vi "MatrixB_Tdep.vi"(0 "T-table String":string, 3 "Time Stamp":timestamp, 6 "Play Button":bool, 7 "Custom Folder":string, 8 "Settings":T2={"Ring 3"=1, "Ring 2"=4, "Fixed Current mkA"=0.5, "If yes, the current is:"=enum."Radio Selection 1", "Ressitance measurements?"=TRUE, "Commute DC current?"=FALSE} {"Ring 3" items=["1 kOhm", "10 kOhm", "100 kOhm", "1 Mohm", "10 mOhm"]; "Ring 2" items=["1 kOhm", "10 kOhm", "100 kOhm", "1 Mohm", "10 MOhm"]}, 9 "Instruments":T3={"Oscillator"=TRUE, "Addr 1 lock-in"=TRUE, "Addr 1 lock-in oop"=TRUE, "Addr 2 lock-in"=TRUE, "Addr 2 lock-in oop"=TRUE, "Addr 3 lock-in"=FALSE, "Addr 3 lock-in oop"=FALSE, "Voltage (Vk1)"=FALSE, "Current (Ik1)"=TRUE, "Voltage (Vk2)"=FALSE, "Current (Ik2)"=FALSE, "Voltage (Vk3)"=FALSE, "Current (Ik3)"=FALSE, "Channel 1 (Vnano1)  "=FALSE, "Channel 2 (Vnano1b)"=FALSE, "Channel 1 (Vnano2)   "=FALSE, "Channel 2 (Vnano2b)"=FALSE, "Thermometer 1 (T1)"=TRUE, "Magnetic Field (B)"=TRUE, "Capacitance (C) and Loss (L)"=FALSE}, 10 "BCluster":T4={"B1 (V)"=-1.0, "B2 (V)"=1.0, "Sweep rate, T/min"=0.5, "Time btw \npoints, sec"=1.0, "No-record rate, T/min"=0.5, "Full sweep?"=FALSE, "Odd confgurations"=TRUE} {"No-record rate, T/min" min=0.0 max=1.0 step=0.01 format="%_4f"; "B2 (V)" min=-4.0 max=4.0 step=0.1 format="%.1f"; "Time btw \npoints, sec" format="%.2f"; "Sweep rate, T/min" min=0.0 max=1.0 step=0.01 format="%_4f"; "B1 (V)" min=-4.0 max=4.0 step=0.1 format="%.1f"}, 11 "TCluster":T1={"Starting T (K)"=-1.0, "Final T (K)"=1.0, "Step (T)"=1.0, "Time for T stabilisation , min"=1.0, "Wait 1st point?"=FALSE, "At the end:"=TRUE} {"Final T (K)" min=-4.0 max=4.0 step=0.1 format="%.2f"; "Time for T stabilisation , min" format="%.2f"; "Step (T)" min=0.0 max=1.0 step=0.01 format="%_4f"; "Starting T (K)" min=-4.0 max=4.0 step=0.1 format="%.2f"}) -> ()   [LabVIEW 2017]
uses:
  <vilib>/Utility/file.llb/Read From Spreadsheet File (DBL).vi
panel:
  in  "No record Vg rate (V/min)":dbl=150.0
  in  "Voltage (sourse)":dbl
  out "Communication":string
  out "B Array":dbl[](array[numeric])
  out "Experiment ends at:":string
  out "Hours":dbl format="%.1f"
  out "Estimated time of experiment:":i16
  out "ArraySens":i8[](array[numeric])
  out "ArrayOsc":dbl[](array[numeric])
  out "# of configurations":i8
  out "Large Array":bool[][][](array[boolean])
  out "Contact configuration file (*.conf)":path
  # "1"
  # "hours"
  # "min.="
  # "Values of T can be also entered as the table by copying\nand pasting a column of numbers in a \"T table\" string at the \nfar right side of this window."
  # "Lock-in Amplifiers"
  # "Temperature"
  # "SourceMeters"
  # "Nanovoltmeters"
  # "Main"
  # "(not recommended, too slow)"
  # "Magnetic Field"
  # "Capacitance & Loss"
  # "(not recommended, too slow)"
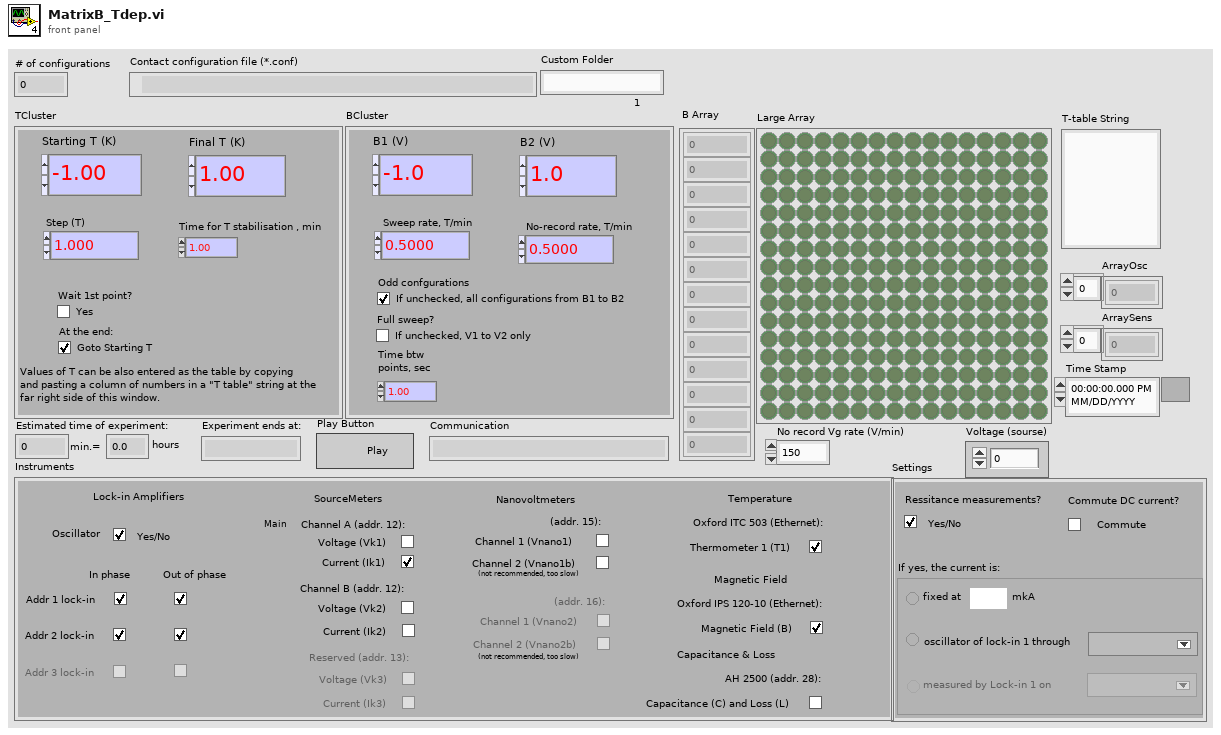
[diagram p1: front panel]
types:
  T1 = cluster{"Starting T (K)":dbl, "Final T (K)":dbl, "Step (T)":dbl, "Time for T stabilisation , min":dbl, "Wait 1st point?":bool, "At the end:":bool}
  T2 = cluster{"Ring 3":u16, "Ring 2":u16, "Fixed Current mkA":dbl, "If yes, the current is:":enum32{"Radio Selection 1", "Radio Selection 2", "Radio Selection 3"}, "Ressitance measurements?":bool, "Commute DC current?":bool}
  T3 = cluster{"Oscillator":bool, "Addr 1 lock-in":bool, "Addr 1 lock-in oop":bool, "Addr 2 lock-in":bool, "Addr 2 lock-in oop":bool, "Addr 3 lock-in":bool, "Addr 3 lock-in oop":bool, "Voltage (Vk1)":bool, "Current (Ik1)":bool, "Voltage (Vk2)":bool, "Current (Ik2)":bool, "Voltage (Vk3)":bool, "Current (Ik3)":bool, "Channel 1 (Vnano1)  ":bool, "Channel 2 (Vnano1b)":bool, "Channel 1 (Vnano2)   ":bool, "Channel 2 (Vnano2b)":bool, "Thermometer 1 (T1)":bool, "Magnetic Field (B)":bool, "Capacitance (C) and Loss (L)":bool}
  T4 = cluster{"B1 (V)":dbl, "B2 (V)":dbl, "Sweep rate, T/min":dbl, "Time btw \npoints, sec":dbl, "No-record rate, T/min":dbl, "Full sweep?":bool, "Odd confgurations":bool}
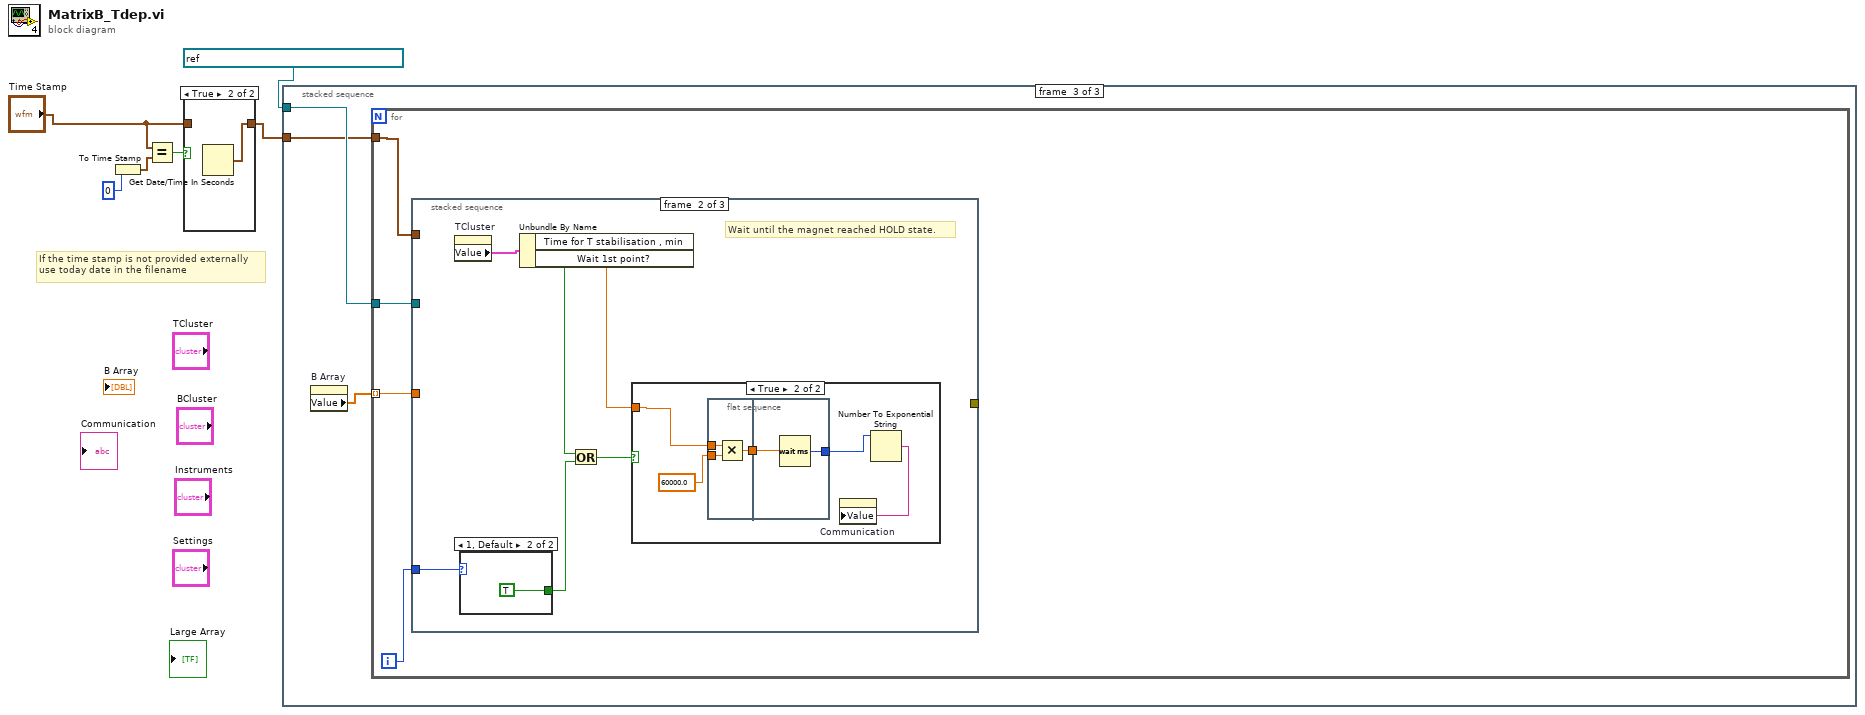
[diagram p0: block diagram]
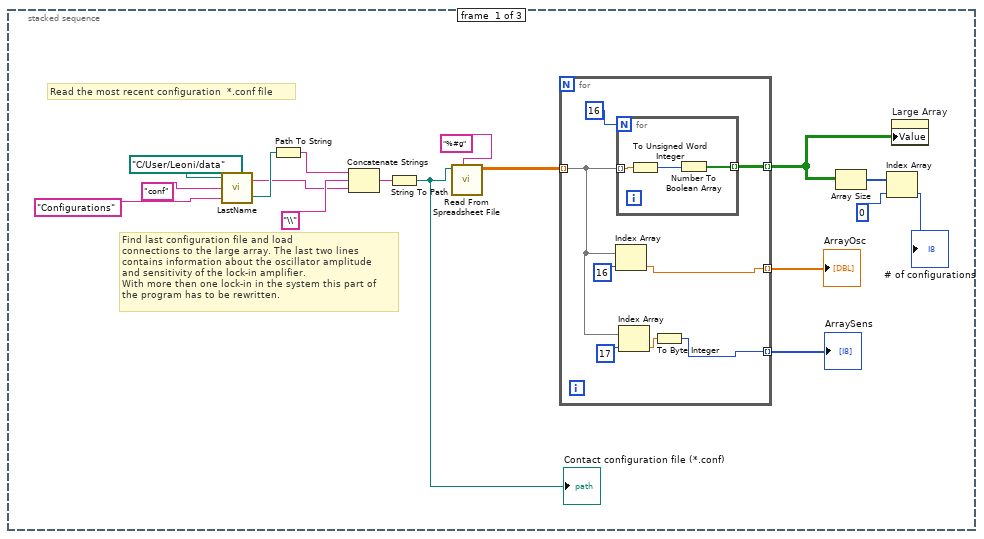
[diagram p3: hidden frame]
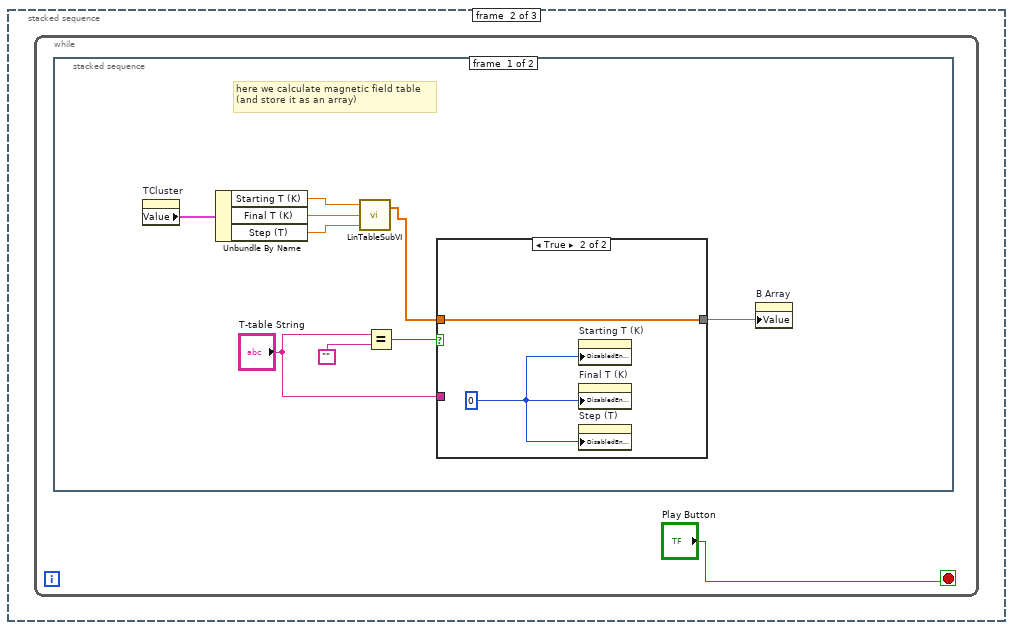
[diagram p4: hidden frame]
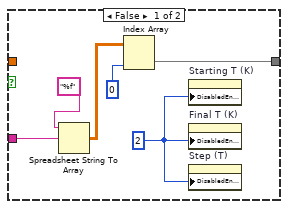
[diagram p5: hidden frame]
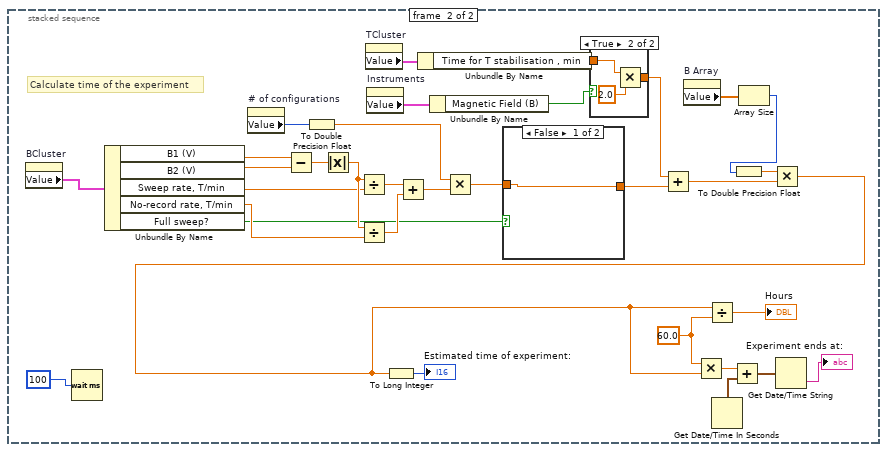
[diagram p6: hidden frame]
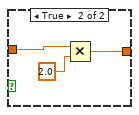
[diagram p8: hidden frame]
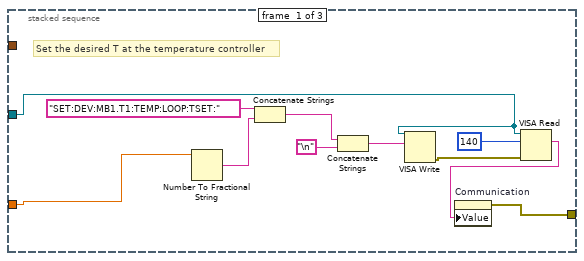
[diagram p9: hidden frame]
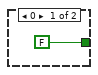
[diagram p11: hidden frame]
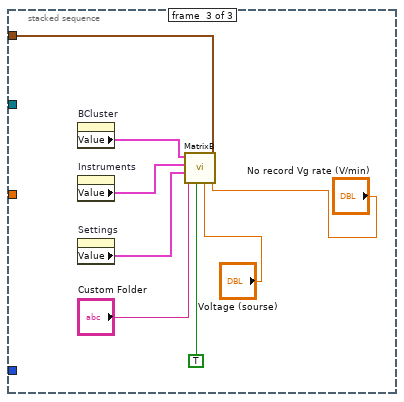
[diagram p12: hidden frame]
diagram:
  # "If the time stamp is not provided externally\nuse today date in the filename"
  n1 = To Time Stamp(1:0) -> (0:w5:timestamp)
  n2 = Equal?(x="Time Stamp", y=w5) -> (x = y?=w4:bool)
  n3 = case shown="True" w4 {
    tunnel: "Time Stamp" -> [w7 _]
    tunnel: [w7 w8] -> w2
    frame False {
    }
    frame True {
      n4 = Get Date/Time In Seconds() -> (seconds since 1Jan1904=w8:timestamp)
    }
  }
  n5 = stacked-sequence {
    tunnel: w2 -> [_ _ w96]
    tunnel: refnum<visa-resource-name> "TCPIP0::192.168.128.2::7020::SOCKET" ("VISA resource name") -> [_ _ w98]
    frame #0 {
      # "Read the most recent configuration  *.conf file"
      # "Find last configuration file and load \nconnections to the large array. The last two lines \ncontains information about the oscillator amplitude\nand sensitivity of the lock-in amplifier.\nWith more then one lock-in in the system this part of \nthe program has to be rewritten."
      n6 = call "LastName.vi"("Custom Folder"="Configurations", "Extention"="conf", "User Data Folder"=path "C:/User/Leoni/data") -> ("created path"=w21:path, "String"=w20:string)
      n7 = Path To String(path=w21) -> (string=w25:string)
      n8 = Concatenate Strings(w25, "\\", w20) -> (w23:string)
      n9 = String To Path(string=w23) -> (path=w11:path)
      "Contact configuration file (*.conf)" <- w11
      n10 = call-poly <vilib>:"Read From Spreadsheet File.vi"("format (%.3f)"="%#g", "file path (dialog if empty)"=w11) -> ("all rows"=w16:dbl[][])  [unwired: 5 in, 4 out]
      n11 = for {
        tunnel: w16 -> [w29] mode=indexing
        tunnel: [w33] -> w13 mode=indexing
        tunnel: [w28] -> w10 mode=indexing
        tunnel: [w27] -> w9 mode=indexing
        n12 = Index Array(array=w29, index=16) -> (element=w28:dbl)
        n13 = for {
          N: 16 -> [_]
          tunnel: w29 -> [w36] mode=indexing
          tunnel: [w34] -> w33 mode=indexing
          n14 = To Unsigned Word Integer(number=w36) -> (unsigned 16bit integer=w35:u16)
          n15 = Number To Boolean Array(number=w35) -> (Boolean array=w34:bool[])
        }
        n16 = Index Array(array=w29, index=17) -> (element=w30:dbl)
        n17 = To Byte Integer(number=w30) -> (8bit integer=w27:i8)
      }
      "ArrayOsc" <- w10
      "ArraySens" <- w9
      n18 = Array Size(array=w13) -> (size(s)=w15:i32[])
      n19 = Index Array(array=w15, index=0) -> (element=→"# of configurations":i32)
      n20 = property on="Large Array" class="Arr (strict)"("Value"=w13) -> ()  [unwired: 2 in, 2 out]
    }
    frame #1 {
      n21 = while {
        stop <- "Play Button" stop-if-true
        n22 = stacked-sequence {
          frame #0 {
            # "here we calculate magnetic field table\n(and store it as an array)"
            n23 = property on="TCluster" class="Clust (strict)"() -> ("Value"=w42:T1)  [unwired: 2 in, 2 out]
            n24 = Unbundle By Name(w42) -> ("Starting T (K)"=w41:dbl, "Final T (K)"=w40:dbl, "Step (T)"=w39:dbl)
            n25 = call "LinTableSubVI.vi"("Step"=w39, "Final"=w40, "Initial"=w41) -> ("Array"=w46:dbl[])  [unwired: 1 in]
            n26 = Equal?(x="T-table String", y="") -> (x = y?=w43:bool)
            n27 = case shown="True" w43 {
              tunnel: [w49 w54] -> w38
              tunnel: w46 -> [_ w54]
              tunnel: "T-table String" -> [w48 _]
              frame False {
                w47 = 2
                n28 = Spreadsheet String To Array(format string="%f", spreadsheet string=w48) -> (array=w51:dbl[][])  [unwired: 2 in]
                n29 = Index Array(array=w51, index (col)=0) -> (element=w49:dbl[])  [unwired: 1 in]
                n30 = property on="Starting T (K)" class="DigNum (strict)"("DisabledEnum"=w47) -> ()  [unwired: 2 in, 2 out]
                n31 = property on="Final T (K)" class="DigNum (strict)"("DisabledEnum"=w47) -> ()  [unwired: 2 in, 2 out]
                n32 = property on="Step (T)" class="DigNum (strict)"("DisabledEnum"=w47) -> ()  [unwired: 2 in, 2 out]
              }
              frame True {
                w53 = 0
                n33 = property on="Starting T (K)" class="DigNum (strict)"("DisabledEnum"=w53) -> ()  [unwired: 2 in, 2 out]
                n34 = property on="Final T (K)" class="DigNum (strict)"("DisabledEnum"=w53) -> ()  [unwired: 2 in, 2 out]
                n35 = property on="Step (T)" class="DigNum (strict)"("DisabledEnum"=w53) -> ()  [unwired: 2 in, 2 out]
              }
            }
            n36 = property on="B Array" class="Arr (strict)"("Value"=w38) -> ()  [unwired: 2 in, 2 out]
          }
          frame #1 {
            w67 = 60.0
            # "Calculate time of the experiment"
            n37 = property on="BCluster" class="Clust (strict)"() -> ("Value"=w86:T4)  [unwired: 2 in, 2 out]
            n38 = Wait (ms)(milliseconds to wait=100) -> ()  [unwired: 1 out]
            n39 = Unbundle By Name(w86) -> ("B1 (V)"=w85:dbl, "B2 (V)"=w84:dbl, "Sweep rate, T/min"=w81:dbl, "No-record rate, T/min"=w80:dbl, "Full sweep?"=w74:bool)
            n40 = property on="# of configurations" class="DigNum (strict)"() -> ("Value"=w76:i8)  [unwired: 2 in, 2 out]
            n41 = Subtract(x=w85, y=w84) -> (x-y=w83:dbl)
            n42 = To Double Precision Float(number=w76) -> (double precision float=w75:dbl)
            n43 = Absolute Value(x=w83) -> (abs(x)=w82:dbl)
            n44 = Divide(x=w82, y=w81) -> (x/y=w79:dbl)
            n45 = Divide(x=w82, y=w80) -> (x/y=w78:dbl)
            n46 = property on="TCluster" class="Clust (strict)"() -> ("Value"=w63:T1)  [unwired: 2 in, 2 out]
            n47 = property on="Instruments" class="Clust (strict)"() -> ("Value"=w58:T3)  [unwired: 2 in, 2 out]
            n48 = Add(x=w79, y=w78) -> (x+y=w77:dbl)
            n49 = Unbundle By Name(w63) -> ("Time for T stabilisation , min"=w56:dbl)
            n50 = Unbundle By Name(w58) -> ("Magnetic Field (B)"=w57:bool)
            n51 = Multiply(x=w75, y=w77) -> (x*y=w73:dbl)
            n52 = case shown="False" w74 {
              tunnel: w73 -> [w92 w95]
              tunnel: [w92 w93] -> w64
              frame False {
              }
              frame True {
                n53 = Multiply(x=w95, y=2.0) -> (x*y=w93:dbl)
              }
            }
            n54 = case shown="True" w57 {
              tunnel: w56 -> [w88 w90]
              tunnel: [w88 w89] -> w55
              frame False {
              }
              frame True {
                n55 = Multiply(x=w90, y=2.0) -> (x*y=w89:dbl)
              }
            }
            n56 = Add(x=w55, y=w64) -> (x+y=w62:dbl)
            n57 = property on="B Array" class="Arr (strict)"() -> ("Value"=w65:dbl[])  [unwired: 2 in, 2 out]
            n58 = Get Date/Time In Seconds() -> (seconds since 1Jan1904=w71:timestamp)
            n59 = Array Size(array=w65) -> (size(s)=w60:i32)
            n60 = To Double Precision Float(number=w60) -> (double precision float=w61:dbl)
            n61 = Multiply(x=w61, y=w62) -> (x*y=w59:dbl)
            n62 = To Long Integer(number=w59) -> (32bit integer=→"Estimated time of experiment:":i32)
            n63 = Multiply(x=w67, y=w59) -> (x*y=w66:dbl)
            n64 = Divide(x=w59, y=w67) -> (x/y=→"Hours":dbl)
            n65 = Add(x=w66, y=w71) -> (x+y=w70:timestamp)
            n66 = Get Date/Time String(seconds (now)=w70) -> (time string=→"Experiment ends at:":string)  [unwired: 2 in, 1 out]
          }
        }
      }
    }
    frame #2 {
      n67 = property on="B Array" class="Arr (strict)"() -> ("Value"=w97:dbl[])  [unwired: 2 in, 2 out]
      n68 = for {
        tunnel: w98 -> [w102]
        tunnel: w97 -> [w101] mode=indexing
        tunnel: w96 -> [w99]
        i -> [w100]
        n69 = stacked-sequence {
          tunnel: w102 -> [w105 _ _]
          tunnel: w101 -> [w103 _ _]
          tunnel: [w113 _ _] -> _
          tunnel: w100 -> [_ w117 _]
          tunnel: w99 -> [_ _ w132]
          frame #0 {
            # "Set the desired T at the temperature controller"
            n70 = Number To Fractional String(number=w103) -> (F-format string=w111:string)  [unwired: 3 in]
            n71 = Concatenate Strings("SET:DEV:MB1.T1:TEMP:LOOP:TSET:" ("string"), w111) -> (w106:string)
            n72 = Concatenate Strings(w106, "\n") -> (w107:string)
            n73 = VISA Write(VISA resource name=w105, write buffer=w107) -> (error out=w110:errorcluster)  [unwired: 1 in, 2 out]
            n74 = VISA Read(VISA resource name=w105, byte count=140, error in (no error)=w110) -> (read buffer=w104:string)  [unwired: 3 out]
            n75 = property on="Communication" class="Str"("Value"=w104) -> (error out=w113:errorcluster)  [unwired: 2 in, 1 out]
          }
          frame #1 {
            # "Wait until the magnet reached HOLD state."
            n76 = property on="TCluster" class="Clust (strict)"() -> ("Value"=w119:T1)  [unwired: 2 in, 2 out]
            n77 = case shown="1, Default" w117 {
              tunnel: [FALSE TRUE] -> w115
              frame 0 {
              }
              frame 1, Default {
              }
            }
            n78 = Unbundle By Name(w119) -> ("Time for T stabilisation , min"=w118:dbl, "Wait 1st point?"=w116:bool)
            n79 = Or(x=w116, y=w115) -> (x .or. y?=w114:bool)
            n80 = case shown="True" w114 {
              tunnel: w118 -> [_ w122]
              frame False {
              }
              frame True {
                n81 = flat-sequence {
                  tunnel: w122 -> [w127]
                  tunnel: 60000.0 -> [w126]
                  tunnel: [w125] -> w120
                  tunnel: [w129] -> w123
                  tunnel: w120 -> [w128]
                  frame #0 {
                    n82 = Multiply(x=w127, y=w126) -> (x*y=w125:dbl)
                  }
                  frame #1 {
                    n83 = Wait (ms)(milliseconds to wait=w128) -> (millisecond timer value=w129:u32)
                  }
                }
                n84 = Number To Exponential String(number=w123) -> (E-format string=w124:string)  [unwired: 3 in]
                n85 = property on="Communication" class="Str"("Value"=w124) -> ()  [unwired: 2 in, 2 out]
              }
            }
          }
          frame #2 {
            n86 = property on="BCluster" class="Clust (strict)"() -> ("Value"=w137:T4)  [unwired: 2 in, 2 out]
            n87 = property on="Instruments" class="Clust (strict)"() -> ("Value"=w133:T3)  [unwired: 2 in, 2 out]
            n88 = property on="Settings" class="Clust (strict)"() -> ("Value"=w134:T2)  [unwired: 2 in, 2 out]
            n89 = call "MatrixB.vi"("No record Vg rate (V/min)"="No record Vg rate (V/min)", "Time Stamp"=w132, "Voltage (sourse)"="Voltage (sourse)", "Play Button"=TRUE, "Custom Folder"="Custom Folder", "Settings"=w134, "Instruments"=w133, "BCluster"=w137) -> ()  [unwired: 4 in]
          }
        }
      }
    }
  }
